vi "Index_patterns_.vi"(1 "LUT":i32[](array[numeric]), 2 "All Patterns in":bool[][](array[boolean])) -> (0 "All Patterns out":bool[][](array[boolean]))   [LabVIEW 2020]
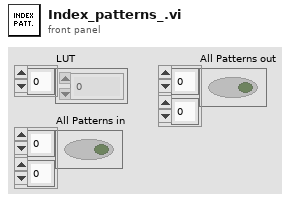
[diagram p1: front panel]
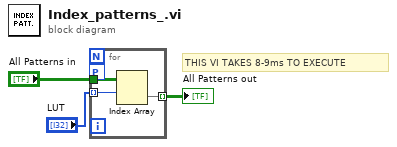
[diagram p0: block diagram]
diagram:
  # "THIS VI TAKES 8-9ms TO EXECUTE"
  n1 = for {
    tunnel: "All Patterns in" -> [w6]
    tunnel: "LUT" -> [w5] mode=indexing
    tunnel: [w4] -> w1 mode=indexing
    workers-P: _ -> [_]
    n2 = Index Array(array=w6, index (row)=w5) -> (element=w4:bool[])  [unwired: 1 in]
  }
  "All Patterns out" <- w1
